vi "CircularBuffer.ImageData.TestLauncher.vi"() -> ()   [LabVIEW 2013, in "CircularBuffer.ImageData.lvclass"]
doc: "JKI State Machine Objects (SMO) 1.0.0.5\nJKI - JKI\nCopyright (c) 2016, JKI"
uses:
  CircularBuffer.ImageData.lvclass
  <vilib>/JKI/JKI SMO/SMO/SMO.lvclass
  CircularBuffer/CircularBuffer.lvclass
  <vilib>/JKI/JKI SMO/SMO/Typedefs/SMOState --Enum.ctl
panel:
  out "BufferSize":i32
  in  "Images":i32(listbox)
  out "Selected Image":picture
  in  "Folder of PNGs":path
  out "State":T1
  out "error out":errorcluster
  in  "Stop":bool
  # "ImageData Buffer Test Launcher"
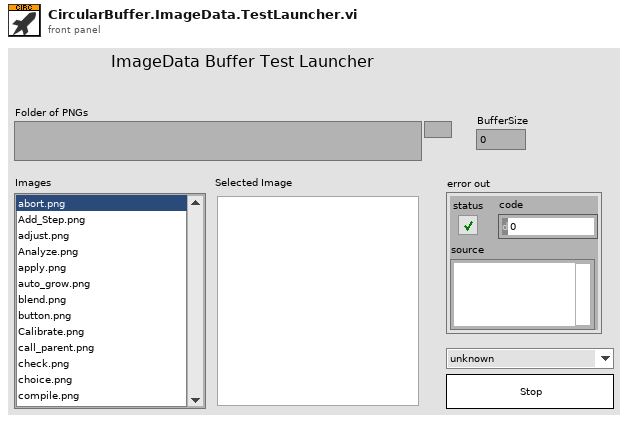
[diagram p1: front panel]
types:
  T1 = typedef "SMO.lvclass/SMOState --Enum.ctl" = enum16{"unknown", "Created", "Started", "Stopped"}
  T2 = typedef "imagedata.ctl" = cluster{"image type":i32, "image depth":i32, "image":u8[], "mask":u8[], "colors":u32[], "Rectangle":cluster{"left":i16, "top":i16, "right":i16, "bottom":i16}}
  T3 = typedef "CircularBuffer.lvclass/PublicEvents--Cluster.ctl" = cluster{"Buffer Resize Event":refnum<user-event>}
  T4 = typedef "SMO.lvclass/Public Events.ctl" = cluster{"Error":refnum<user-event>, "State":refnum<user-event>}
  T5 = cluster{"Event Registration Refnum":refnum<event-registration>}
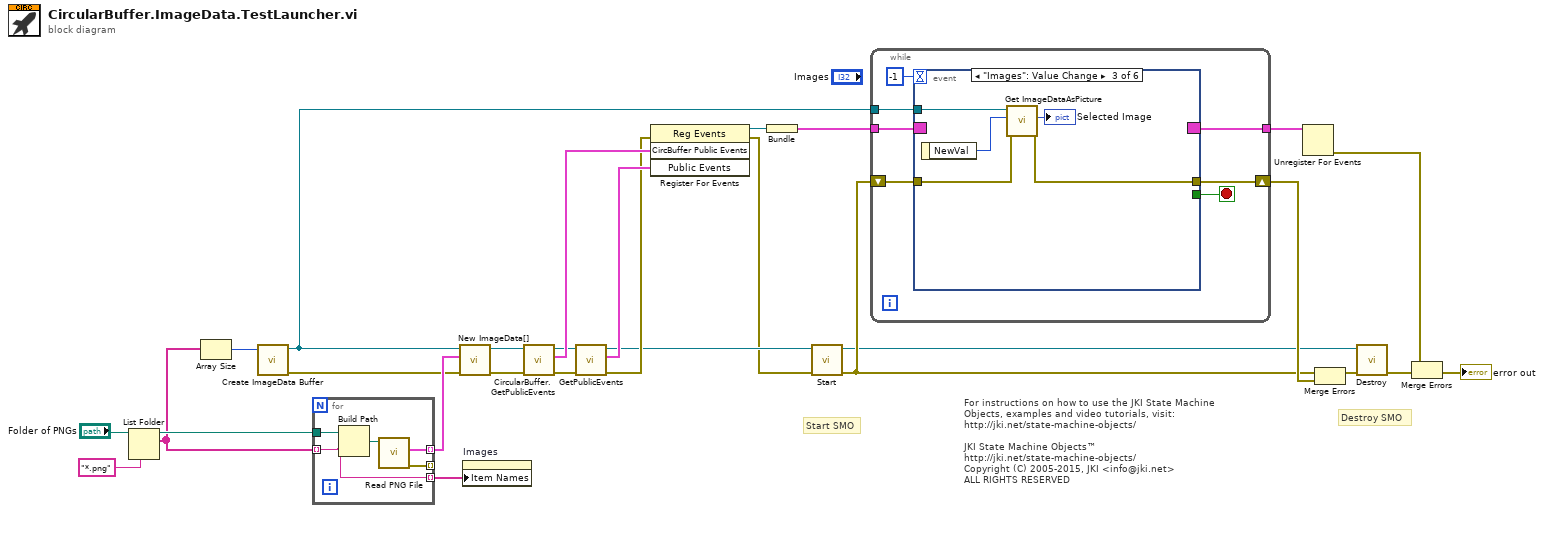
[diagram p0: block diagram]
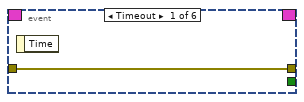
[diagram p2: hidden frame]
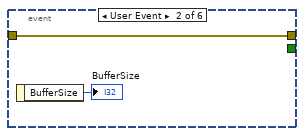
[diagram p3: hidden frame]
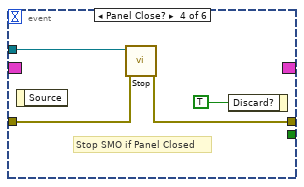
[diagram p4: hidden frame]
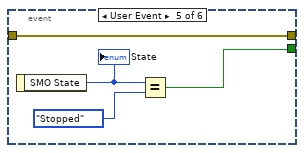
[diagram p5: hidden frame]
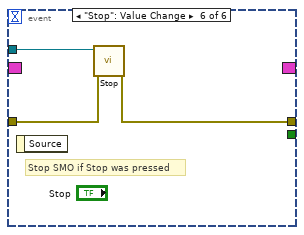
[diagram p6: hidden frame]
diagram:
  # "For instructions on how to use the JKI State Machine Objects, examples and video tutorials, visit:\nhttp://jki.net/state-machine-objects/\n\nJKI State Machine Objects™\nhttp://jki.net/state-machine-objects/\nCopyright (C) 2005-2015, JKI <info@jki.net>\nALL RIGHTS RESERVED"
  # "Start SMO"
  # "Destroy SMO"
  n1 = List Folder(path="Folder of PNGs", pattern="*.png") -> (path out=w9:path, filenames=w8:string[])  [unwired: 2 in, 2 out]
  n2 = Array Size(array=w8) -> (size(s)=w6:i32)
  n3 = call "Create ImageData Buffer.vi"("BufferSize"=w6) -> ("error out"=w1:errorcluster, "CircularBuffer.ImageData out"=w5:refnum<class "CircularBuffer.ImageData.lvclass">)  [unwired: 8 in, 1 out]
  n4 = for {
    tunnel: w9 -> [w33]
    tunnel: w8 -> [w31] mode=indexing
    tunnel: [w31] -> w7 mode=indexing
    tunnel: [w30] -> w4 mode=indexing
    tunnel: [w29] -> _ mode=indexing
    n5 = Build Path(base path=w33, name or relative path=w31) -> (appended path=w32:path)
    n6 = call <vilib>:"Read PNG File.vi"("path to PNG file"=w32) -> ("error out"=w29:errorcluster, "image data"=w30:T2)  [unwired: 8 in, 1 out]
  }
  n7 = call "New ImageData[].vi"("error in (no error)"=w1, "ImageData[]"=w4, "CircularBuffer.ImageData"=w5) -> ("error out"=w2:errorcluster, "CircularBuffer.ImageData out"=w3:refnum<class "CircularBuffer.ImageData.lvclass">)  [unwired: 6 in, 1 out]
  n8 = property on="Images" class="LstBox (strict)"("Item Names"=w7) -> ()  [unwired: 2 in, 2 out]
  n9 = call "CircularBuffer.GetPublicEvents.vi"("error in (no error)"=w2, "CircularBuffer"=w3) -> ("error out"=w18:errorcluster, "CircBuffer Public Events"=w21:T3, "CircularBuffer out"=w19:refnum<class "CircularBuffer.ImageData.lvclass">)  [unwired: 7 in]
  n10 = call <vilib>:"GetPublicEvents.vi"("error in (no error)"=w18, "SMO"=w19) -> ("error out"=w16:errorcluster, "Public Events"=w17:T4, "SMO out"=w13:refnum<class "CircularBuffer.ImageData.lvclass">)  [unwired: 7 in]
  n11 = register-events(error in=w16, w21, w17) -> (reference out=w20:refnum<event-registration>, error out=w12:errorcluster)  [unwired: 1 in]
  n12 = Bundle("Event Registration Refnum"=w20) -> (w27:T5)  [unwired: 1 in]
  n13 = call <vilib>:"Start.vi"("error in (no error)"=w12, "SMO"=w13) -> ("error out"=w22:errorcluster, "SMO out"=w14:refnum<class "CircularBuffer.ImageData.lvclass">)  [unwired: 8 in]
  n14 = while {
    shift-right: [w39] -> w26
    shift-left: w22 -> [w38]
    tunnel: w27 -> [w37]
    tunnel: [w36] -> w28
    tunnel: w5 -> [w35]
    stop <- w40 stop-if-true
    n15 = event shown="[2] \"Images\": Value Change" {
      selector: w37 -> [_ _ _ _ _ _]
      dyn-events: [_ _ _ _ _ _] -> w36
      timeout: -1 -> [_ _ _ _ _ _]
      tunnel: [_ _ _ _ w53 _] -> w40
      tunnel: w35 -> [_ _ w48 w52 _ w59]
      tunnel: [w41 w43 w47 w51 w56 w58] -> w39
      tunnel: w38 -> [w41 w43 w45 w50 w56 w57]
      event Timeout {
        n16 = event-data() -> ()  [unwired: 1 in, 1 out]
      }
      event User Event {
        n17 = event-data() -> ("BufferSize"=→"BufferSize":i32)  [unwired: 1 in]
      }
      event "Images": Value Change {
        n18 = event-data() -> ("NewVal"=w44:i32)  [unwired: 1 in]
        n19 = call "Get ImageDataAsPicture.vi"("error in (no error)"=w45, "GetElement (-1: Current)"=w44, "CircularBuffer.ImageData"=w48) -> ("error out"=w47:errorcluster, "Selected Image"=→"Selected Image":picture)  [unwired: 6 in, 1 out]
      }
      event Panel Close? {
        # "Stop SMO if Panel Closed"
        n20 = event-data() -> ()  [unwired: 1 in, 1 out]
        n21 = call <vilib>:"Stop.vi"("error in (no error)"=w50, "SMO"=w52) -> ("error out"=w51:errorcluster)  [unwired: 8 in, 1 out]
        n22 = event-data("Discard?"=TRUE ("OK")) -> ()  [unwired: 1 in, 1 out]
      }
      event User Event {
        n23 = event-data() -> ("SMO State"=w55:T1)  [unwired: 1 in]
        "State" <- w55
        n24 = Equal?(x=w55, y=SMOState_--Enum."Stopped") -> (x = y?=w53:bool)
      }
      event "Stop": Value Change {
        # "Stop SMO if Stop was pressed"
        n25 = event-data() -> ()  [unwired: 1 in, 1 out]
        n26 = call <vilib>:"Stop.vi"("error in (no error)"=w57, "SMO"=w59) -> ("error out"=w58:errorcluster)  [unwired: 8 in, 1 out]
      }
    }
  }
  n27 = Unregister For Events(event registration refnum=w28) -> (error out=w25:errorcluster)  [unwired: 1 in]
  n28 = Merge Errors(w22, w26) -> (w15:errorcluster)
  n29 = call <vilib>:"Destroy.vi"("error in (no error)"=w15, "SMO"=w14) -> ("error out"=w23:errorcluster)  [unwired: 9 in]
  n30 = Merge Errors(w25, w23) -> (→"error out":errorcluster)
